vi "GUI Test Chennels.vi"() -> ()   [LabVIEW 2019]
panel:
  out "Vertical Fill Indicator 2":dbl(slide)=5.954198473282443 caption="Температура масла" scale=0.0..10.0
  out "Уровень  масла 2":dbl(slide)=37.72455089820359 caption="Уровень  масла" scale=0.0..100.0
  out "Vertical Fill Indicator":dbl(slide)=5.954198473282443 caption="Температура масла" scale=0.0..10.0
  out "Уровень  масла":dbl(slide)=37.72455089820359 scale=0.0..100.0
  out "DI 17":bool caption="Источник\nпитания 24 В"
  out "DI 9":bool caption="Реле контроля фаз \nКонтактор"
  out "DI 11":bool caption="QF5"
  out "DI 10":bool caption="QF4"
  out "DI 8":bool caption="QF3"
  out "DI 7":bool caption="QF2"
  out "DI 6":bool caption="QF1"
  out "DI 5":bool caption="Автомат"
  out "DI 4":bool caption="Контактор"
  out "DI 3":bool caption="Автомат"
  out "DI 2":bool caption="Контактор"
  out "DI 1":bool caption="Автомат"
  out "DI 0":bool caption="Контактор"
  in  "AO 1":dbl(slide)=1.0 caption="AO 0" scale=0.0..10.0
  in  "AO 0":dbl(slide)=1.0 scale=0.0..10.0
  in  "DO 16":bool caption="KP17"
  in  "DO 15":bool caption="KP16"
  in  "DO 14":bool caption="KP15"
  in  "DO 13":bool caption="KP14"
  in  "DO 12":bool caption="KP13"
  in  "DO 11":bool caption="KP12"
  in  "DO 10":bool caption="KP11"
  in  "DO 9":bool caption="KP10"
  in  "DO 8":bool caption="KP9"
  in  "DO 7":bool caption="KP8"
  in  "DO 6":bool caption="KP7"
  in  "DO 5":bool caption="KP6"
  in  "DO 4":bool caption="KP5"
  in  "DO 3":bool caption="KP4"
  in  "DO 2":bool caption="KP3 [DO 2]"
  in  "DO 1":bool caption="KP2 [DO 1]"
  in  "DO 0":bool caption="KP1 [DO 0]"
  out "DI 16":bool caption="Переключатель ручное/авто SA1"
  out "DI 15":bool caption="Кнопка аварийной остановки SB4"
  out "DI 14":bool caption="Кнопка остановки SB3"
  out "DI 13":bool caption="Кнопка запуска SB2"
  out "DI 12":bool caption="Кнопка сброса ошибки SB1"
  out "Gauge 11":dbl(knob) caption="Датчик давления в линии \nизмерения утечек" scale=0.0..10.0
  out "Gauge 10":dbl(knob) caption="Давление  в  линии подачи \nвоздуха после БПВ" scale=0.0..10.0
  out "Gauge 9":dbl(knob) caption="Давление  в  линии подачи \nвоздуха в БПВ" scale=0.0..10.0
  out "Gauge 8":dbl(knob) caption="Давление в камере" scale=0.0..10.0
  out "Gauge 7":dbl(knob) caption="Давление в образце" scale=0.0..10.0
  out "Gauge 6":dbl(knob) caption="Давление после насоса ВД" scale=0.0..10.0
  # "Проверка каналов"
  # "Панель гидравлическая"
  # "Реле"
  # "Гидростанция очистки и охлаждения"
  # "Насоса перекачки \nв бак подачи"
  # "PUMP1"
  # "PUMP0"
  # "Гидростанция подачи масла"
  # "Кнопки"
  # "Автоматы"
  # "PUMP2"
  # "Управление  подачей давления в насос ВД"
  # "Ethernet Devices"
  # "Регулировка низкого давления в линии подачи масла в насос ВД и напрямую в узел образца"
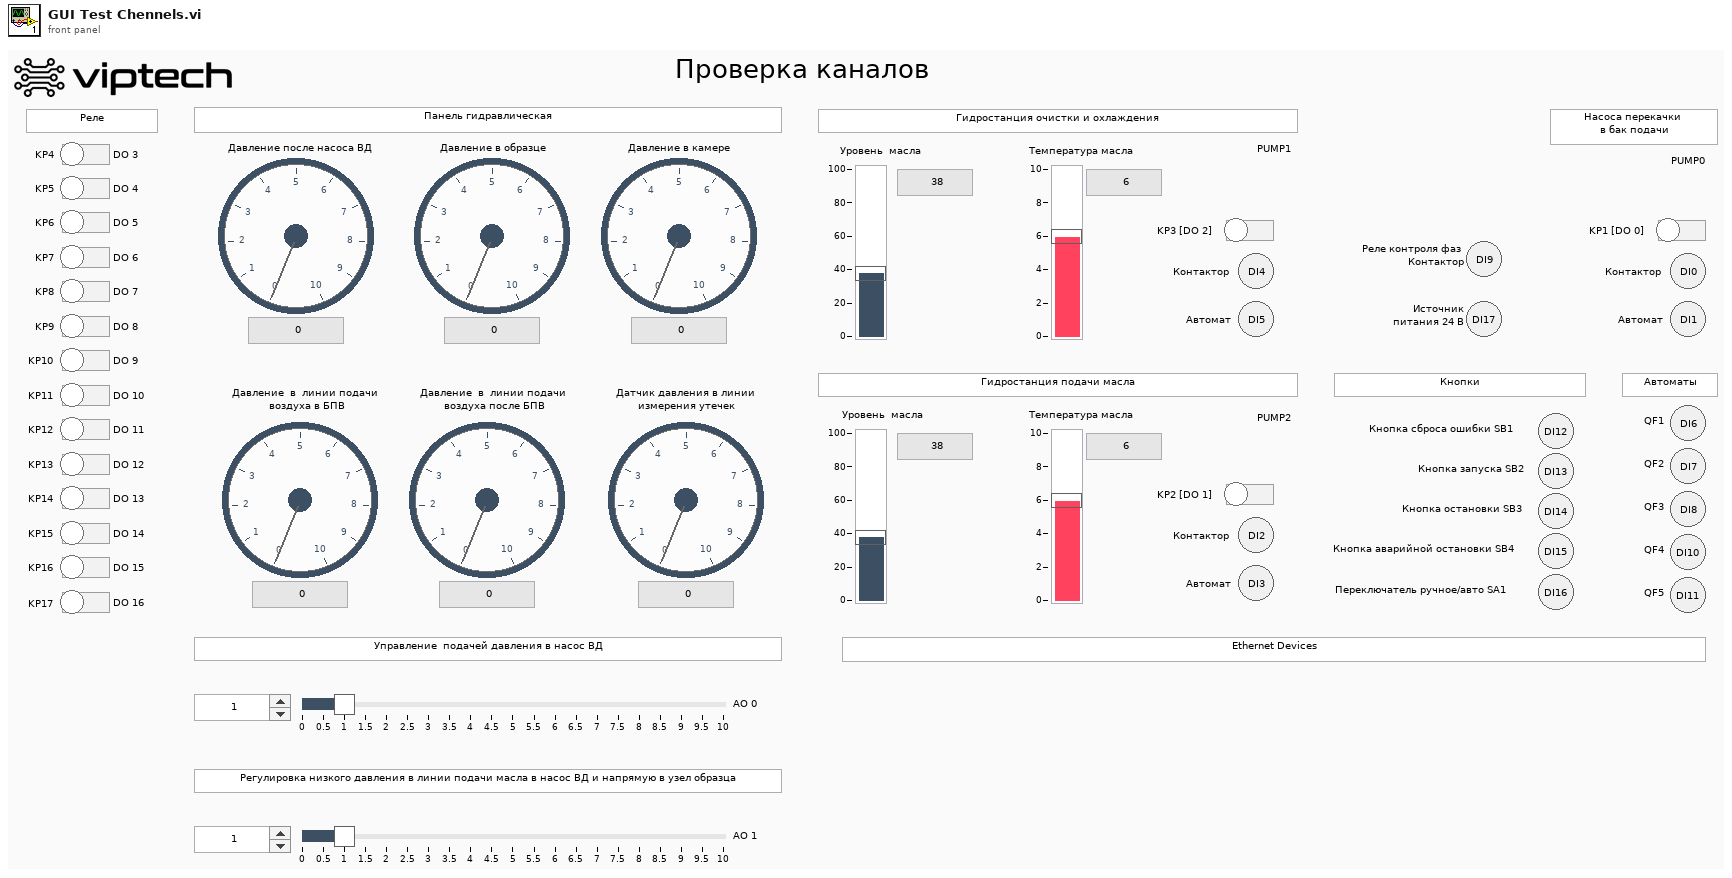
[diagram p1: front panel]
types:
  T1 = enum32{"Invalid", "Standard", "Closed", "Hidden", "Minimized", "Maximized"}
  T2 = enum32{"invalid app kind", "Development System", "Run Time System", "Student Edition", "Embedded LabVIEW", "Evaluation", "Custom"}
  T3 = cluster{"Core":cluster{"Current VI Reference":refnum<vi>, "Close Panel on Exit?":bool}, "Your Boolean data":bool, "Your string data":string}
  T4 = cluster{"Current VI Reference":refnum<vi>, "Close Panel on Exit?":bool}
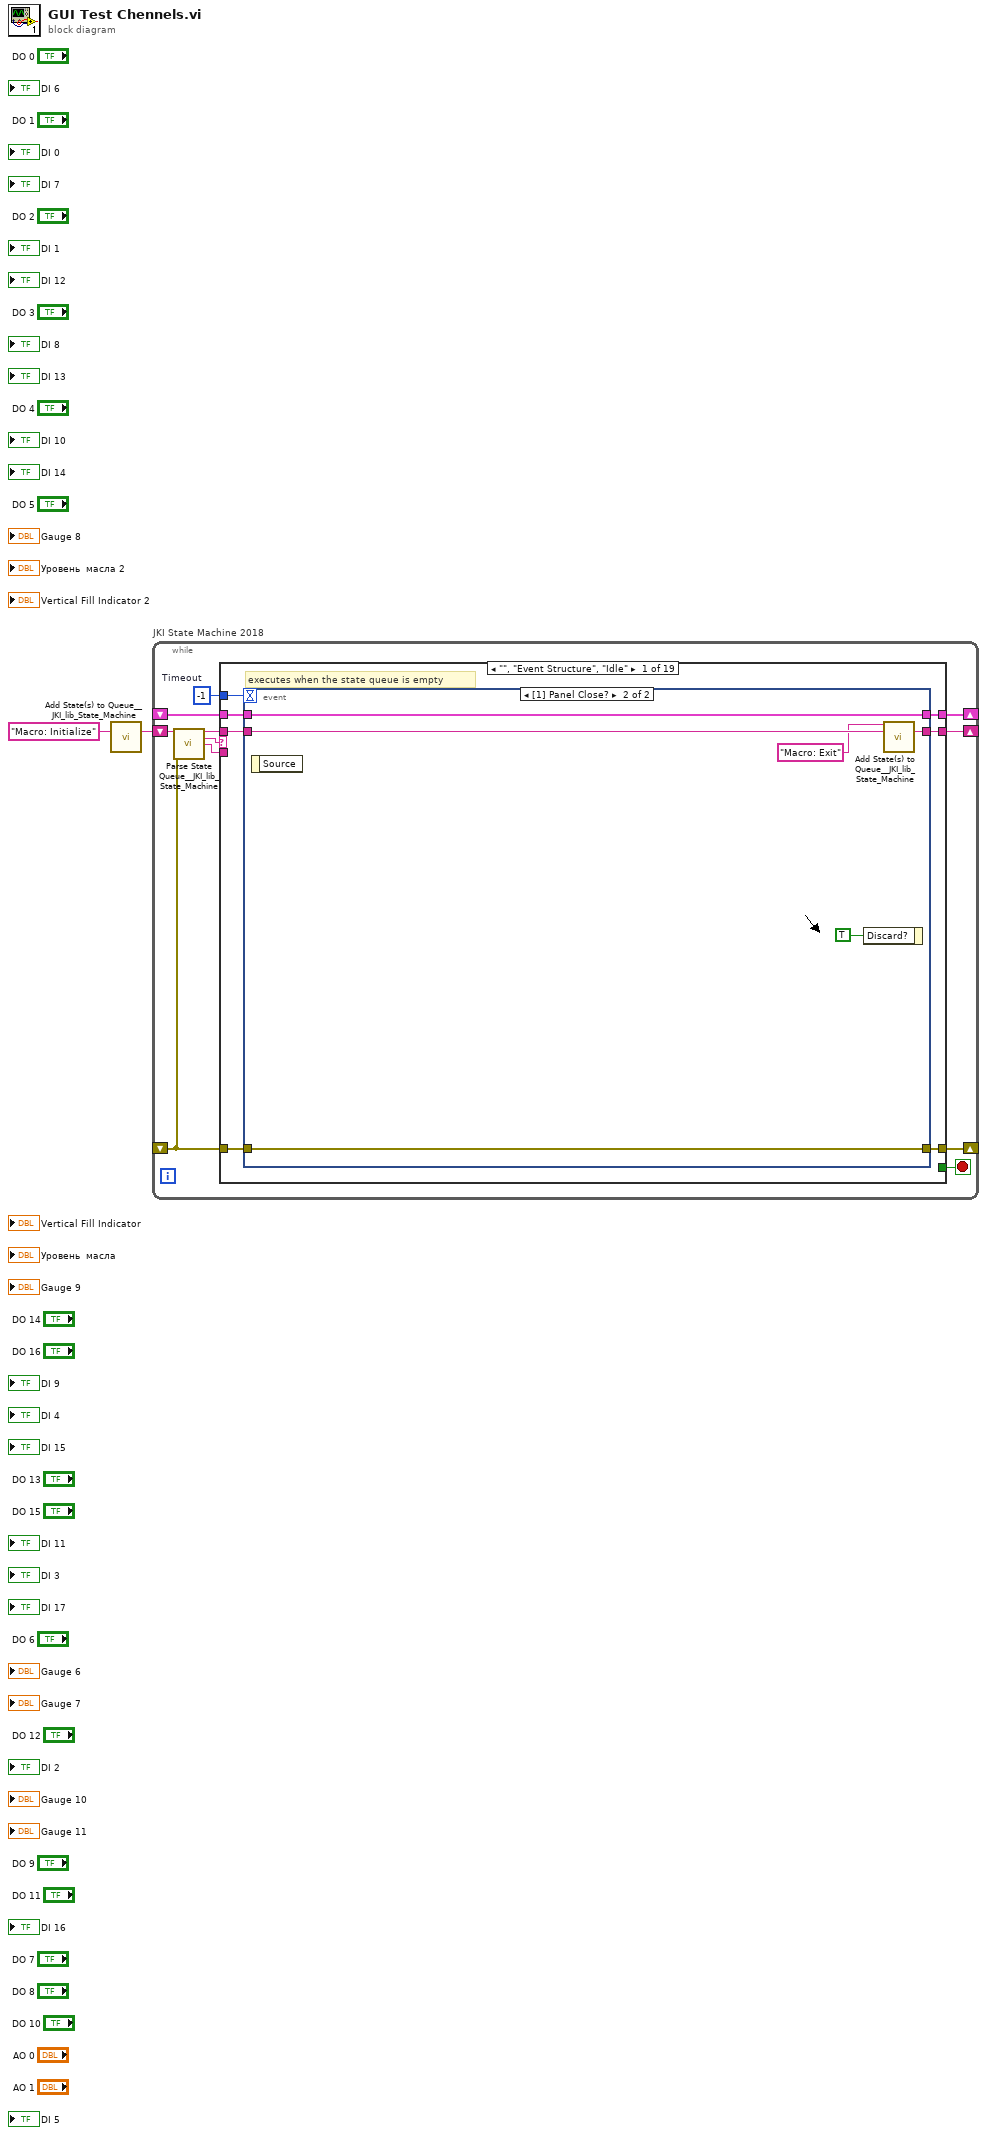
[diagram p0: block diagram]
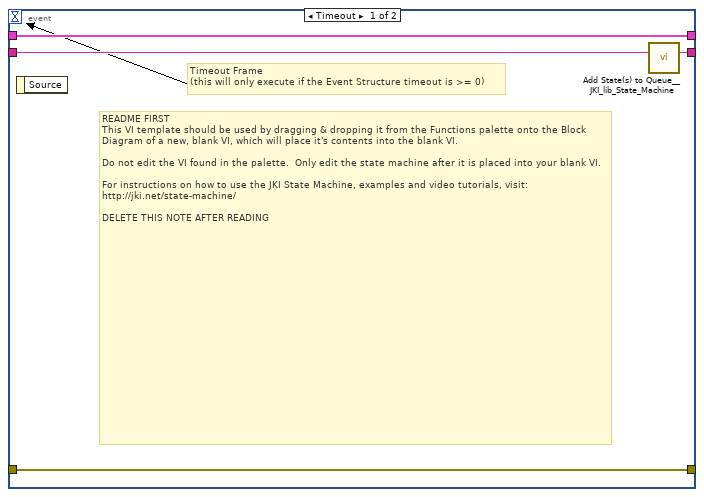
[diagram p2: hidden frame]
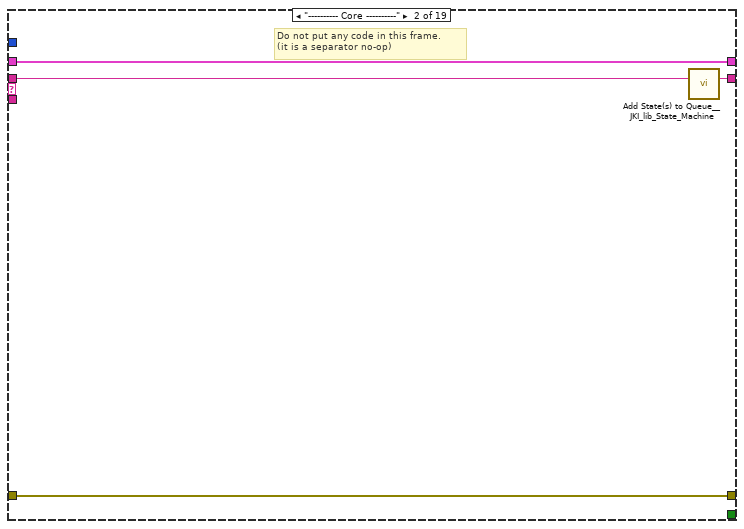
[diagram p3: hidden frame]
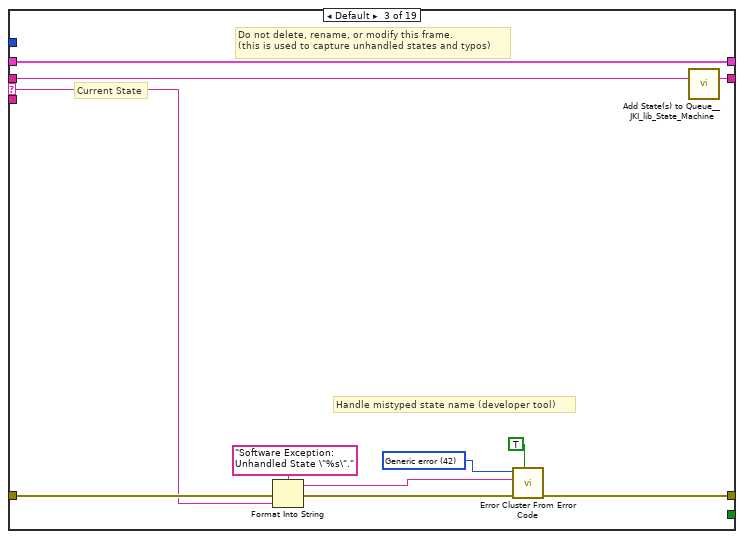
[diagram p4: hidden frame]
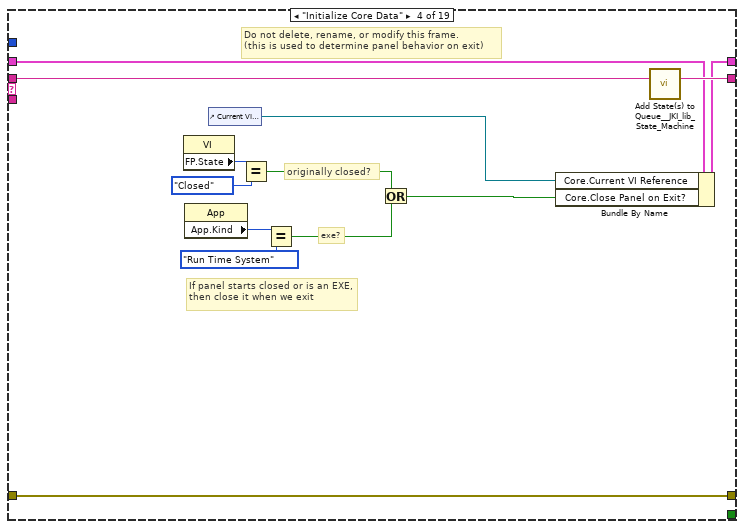
[diagram p5: hidden frame]
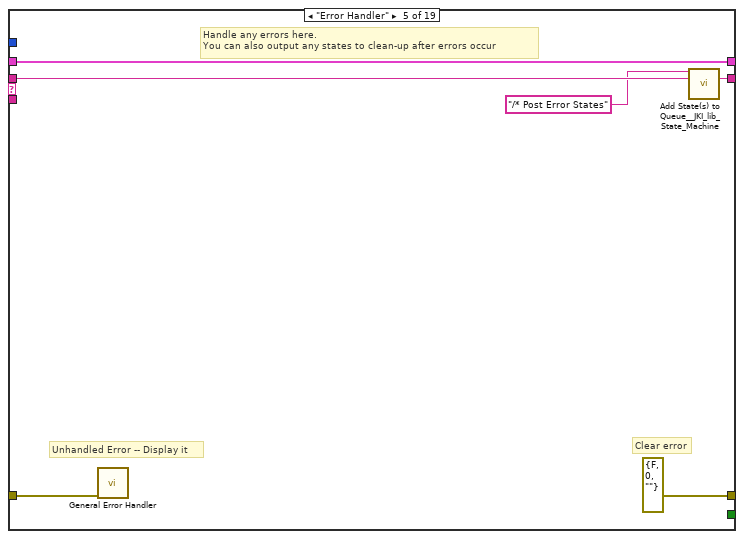
[diagram p6: hidden frame]
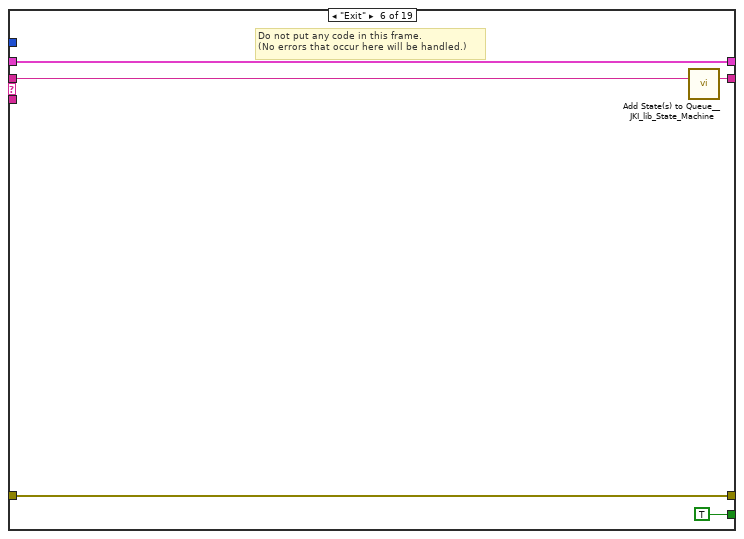
[diagram p7: hidden frame]
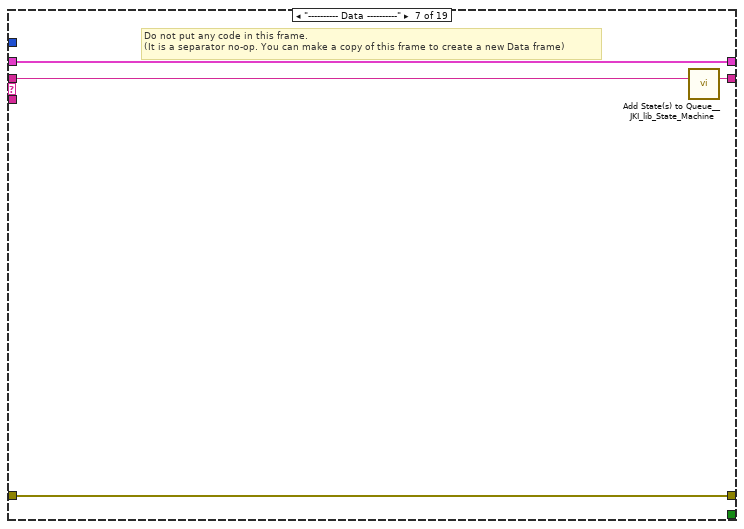
[diagram p8: hidden frame]
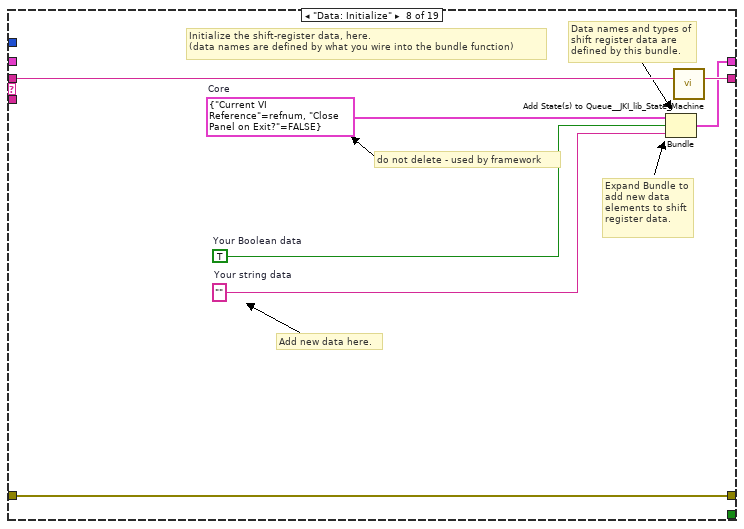
[diagram p9: hidden frame]
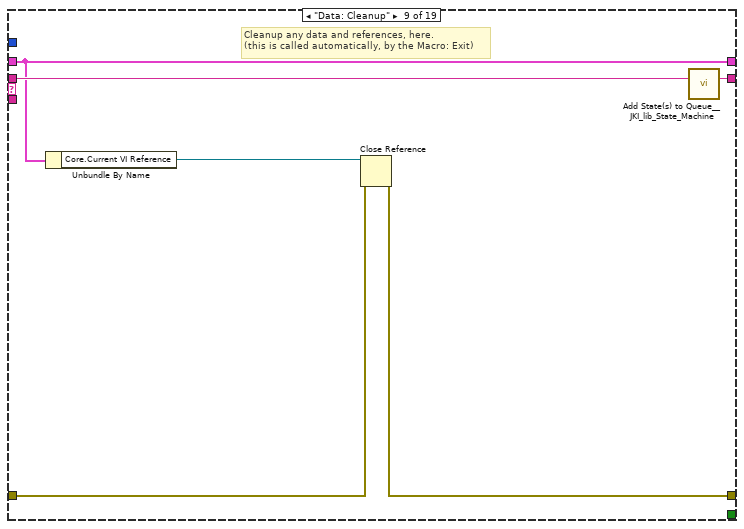
[diagram p10: hidden frame]
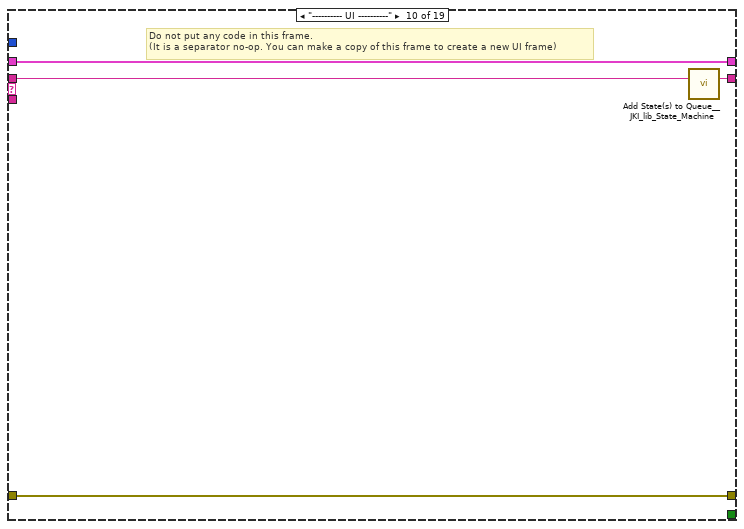
[diagram p11: hidden frame]
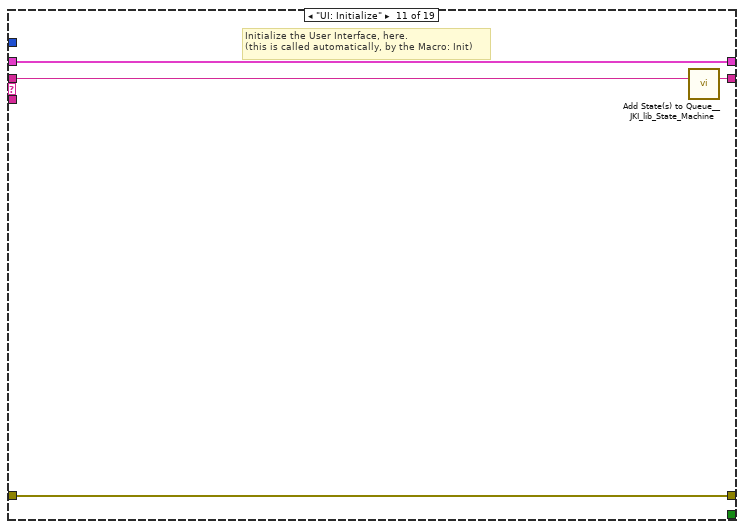
[diagram p12: hidden frame]
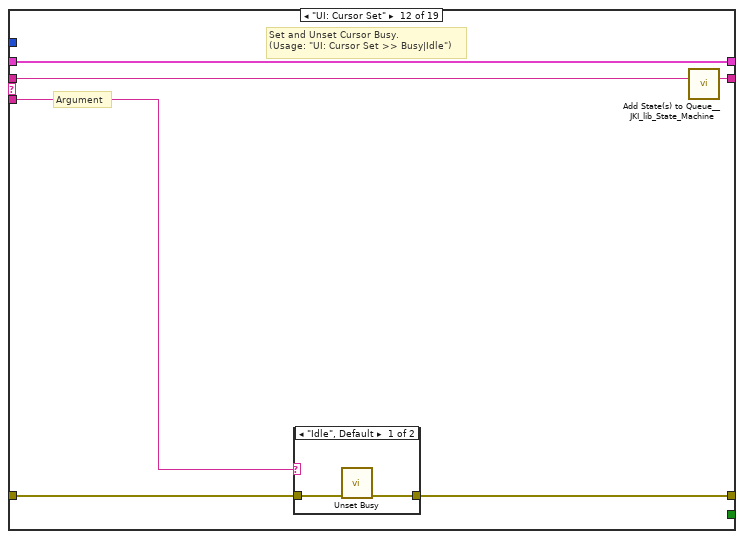
[diagram p13: hidden frame]
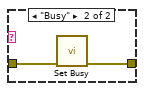
[diagram p14: hidden frame]
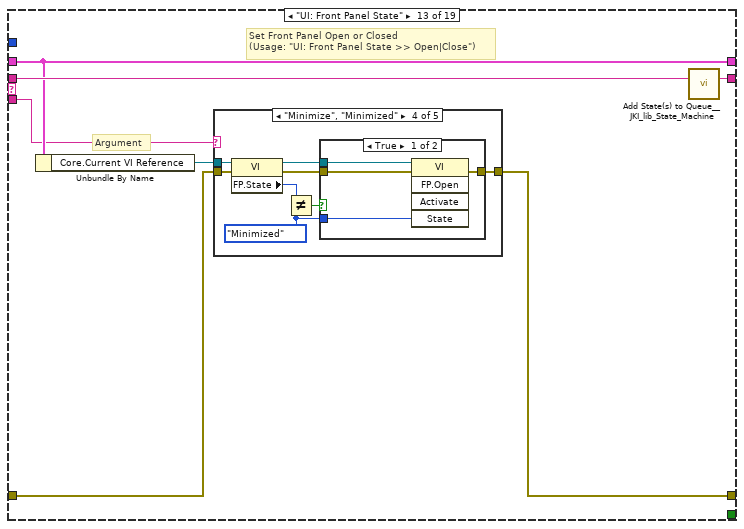
[diagram p15: hidden frame]
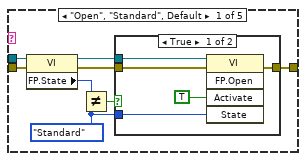
[diagram p16: hidden frame]
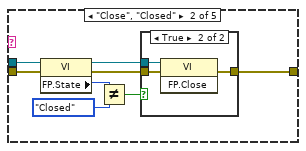
[diagram p18: hidden frame]
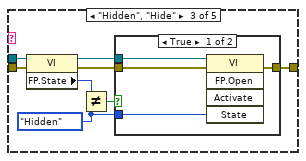
[diagram p20: hidden frame]
diagram:
  n1 = call <vilib>:"Add State(s) to Queue__JKI_lib_State_Machine.vi"("State(s) in (\"\")"="Macro: Initialize") -> ("States Out"=w2:string)  [unwired: 14 in]
  n2 = while "JKI State Machine 2018" {
    shift-right: [w6] -> _
    shift-left: _ -> [w5]
    shift-right: [w9] -> _
    shift-left: _ -> [w3]
    shift-right: [w8] -> _
    shift-left: w2 -> [w10]
    stop <- w7 stop-if-true
    w4 = -1  # Timeout
    n3 = call <vilib>:"Parse State Queue__JKI_lib_State_Machine.vi"("State Queue"=w10, "Error In (no error)"=w3) -> ("Remaining States"=w12:string, "Current State"=w13:string, "Arguments"=w11:string)  [unwired: 11 in]
    n4 = case shown="\"\", \"Event Structure\", \"Idle\"" w13 {
      selector: w13 -> [_ _ w35 _ _ _ _ _ _ _ _ _ _ _ _ _ _ _ _]
      tunnel: w12 -> [w20 w34 w39 w58 w64 w69 w73 w80 w86 w90 w94 w100 w111 w180 w185 w195 w199 w203 w207]
      tunnel: w11 -> [_ _ _ _ _ _ _ _ _ _ _ w95 w105 _ _ _ _ _ _]
      tunnel: w5 -> [w18 w31 w37 w51 w61 w67 w70 _ w81 w87 w92 w98 w107 w177 w182 w192 w196 w200 w204]
      tunnel: [w17 w32 w41 w55 errorcluster {"status"=FALSE, "code"=0, "source"=""} ("error out") w66 w71 w77 w82 w88 w91 w96 w108 w178 w183 w193 w197 w201 w205] -> w9
      tunnel: w3 -> [w16 w32 w40 w55 w60 w66 w71 w77 w83 w88 w91 w97 w109 w178 w183 w193 w197 w201 w205]
      tunnel: [w19 w33 w38 w57 w63 w68 w72 w79 w85 w89 w93 w99 w110 w179 w184 w194 w198 w202 w206] -> w8
      tunnel: [_ _ _ _ _ TRUE _ _ _ _ _ _ _ _ _ _ _ _ _] -> w7
      tunnel: [w15 w31 w37 w56 w61 w67 w70 w78 w81 w87 w92 w98 w107 w177 w182 w192 w196 w200 w204] -> w6
      tunnel: w4 -> [w14 _ _ _ _ _ _ _ _ _ _ _ _ _ _ _ _ _ _]
      frame "", "Event Structure", "Idle" {
        # "executes when the state queue is empty"
        n5 = event shown="[1] Panel Close?" {
          selector: _ -> [_ _]
          dyn-events: _ -> [_ _]
          timeout: w14 -> [_ _]
          tunnel: w20 -> [w24 w30]
          tunnel: [w23 w29] -> w19
          tunnel: w18 -> [w21 w27]
          tunnel: [w22 w28] -> w17
          tunnel: w16 -> [w22 w28]
          tunnel: [w21 w27] -> w15
          event Timeout {
            # "README FIRST\nThis VI template should be used by dragging & dropping it from the Functions palette onto the Block Diagram of a new, blank VI, which will place it's contents into the blank VI.\n\nDo not edit the VI found in the palette.  Only edit the state machine after it is placed into your blank VI.\n\nFor instructions on how to use the JKI State Machine, examples and video tutorials, visit:\nhttp://jki.net/state-machine/\n\nDELETE THIS NOTE AFTER READING"
            # "Timeout Frame\n(this will only execute if the Event Structure timeout is >= 0)"
            n6 = event-data() -> ()  [unwired: 1 in, 1 out]
            n7 = call <vilib>:"Add State(s) to Queue__JKI_lib_State_Machine.vi"("State(s) in (\"\")"=w24) -> ("States Out"=w23:string)  [unwired: 14 in]
          }
          event Panel Close? {
            n8 = event-data() -> ()  [unwired: 1 in, 1 out]
            n9 = event-data("Discard?"=TRUE) -> ()  [unwired: 1 in, 1 out]
            n10 = call <vilib>:"Add State(s) to Queue__JKI_lib_State_Machine.vi"("State(s) in Front (\"\")"="Macro: Exit", "State(s) in (\"\")"=w30) -> ("States Out"=w29:string)  [unwired: 13 in]
          }
        }
      }
      frame "---------- Core ----------" {
        # "Do not put any code in this frame.\n(it is a separator no-op)"
        n11 = call <vilib>:"Add State(s) to Queue__JKI_lib_State_Machine.vi"("State(s) in (\"\")"=w34) -> ("States Out"=w33:string)  [unwired: 14 in]
      }
      frame Default {
        w44 = 42 items=["No error", "Argument error", "Memory is full", "Out of zone", "End of file", "File already open", "Generic file I/O error", "File not found", "File permission error", "Disk is full", "Duplicate path", "Too many files open", "System feature not enabled", "Resource file not found", "Cannot add resource", "Resource not found", "Image not found", "Image memory error", "Pen does not exist", "Config type invalid", "Config token not found", "Config parse error", "Config memory error", "Bad external code format", "Bad external code offset", "External code not present", "Null window", "Destroy window error", "Null menu", "Print aborted", "Bad print record", "Print driver error", "Windows error during printing", "Memory error during printing", "Print dialog error", "Generic print error", "Invalid device refnum", "Device not found", "Device parameter error", "Device unit error", "Cannot open device", "Device call aborted", "Generic error", "Cancelled by user", "Object ID too low", "Object ID too high", "Object not in heap", "Unknown heap", "Unknown object (invalid DefProc)", "Unknown object (DefProc not in table)", "Message out of range", "Invalid (null) method", "Unknown message", "Manager call not supported", "Bad address", "Network operation in progress", "Network operation timed out", "Connection is busy", "Network attribute not supported", "Network error", "Address in use", "System out of memory", "Connection aborted", "Connection refused", "Not connected", "Already connected", "Connection closed", "Initialization error (interapplication manager)", "Bad occurrence", "Wait on unbound occurrence handler", "Occurrence queue overflow", "Datalog type conflict", "Unused", "Unrecognized type (interapplication manager)", "Memory corrupt", "Failed to make temporary DLL", "Old CIN version", "Drag socket not found", "Failed to load drop-object", "Failed to register OLE object", "Failed to release OLE object", "Format specifier type mismatch", "Unknown format specifier", "Too few format specifiers", "Too many format specifiers", "Scan failed", "Newer CIN version", "Error converting to variant", "Runtime menu error", "Password tampered", "Variant attribute not found", "Incompatible variant data type", "Event data is not available", "Event Store is not present", "Occurrence is not found", "Event Queue is not created", "Event info is not available", "Refnum passed is NULL", "Error retrieving Class GUID", "Error retrieving CoClass GUID", "Error retrieving TypeLib GUID.", "Bad built application magic bytes.", "Specific driver is different from the specific driver associated with the Logical Name.", "There is no session opened to the class driver.", "Max Error", "MAX - Error with config objects", "MAX - Error loading configuration", "MAX - Group not supported"]
        # "Current State"
        # "Do not delete, rename, or modify this frame.\n(this is used to capture unhandled states and typos)"
        # "Handle mistyped state name (developer tool)"
        n12 = Format Into String(format string="Software Exception: Unhandled State \"%s\"." ("message"), error in=w40, w35) -> (resulting string=w43:string, error out=w42:errorcluster)  [unwired: 1 in]
        n13 = call <vilib>:"Error Cluster From Error Code.vi"("show call chain? (False)"=TRUE, "error in (no error)"=w42, "error message (\"\")"=w43, "error code (0)"=w44) -> ("error out"=w41:errorcluster)  [unwired: 5 in]
        n14 = call <vilib>:"Add State(s) to Queue__JKI_lib_State_Machine.vi"("State(s) in (\"\")"=w39) -> ("States Out"=w38:string)  [unwired: 14 in]
      }
      frame "Initialize Core Data" {
        # "Do not delete, rename, or modify this frame.\n(this is used to determine panel behavior on exit)"
        # "originally closed?"
        # "exe?"
        # "If panel starts closed or is an EXE, then close it when we exit"
        n15 = property class="VI"() -> ("FP.State"=w48:T1)  [unwired: 2 in, 2 out]
        n16 = property class="App"() -> ("App.Kind"=w54:T2)  [unwired: 2 in, 2 out]
        n17 = control-ref of="Current VI Reference"() -> (w49:refnum<vi>)
        n18 = Equal?(x=w48, y=T1."Closed" ("Front Panel Window:State")) -> (x = y?=w46:bool)
        n19 = Equal?(x=w54, y=T2."Run Time System" ("Application:Kind")) -> (x = y?=w52:bool)
        n20 = Or(x=w46, y=w52) -> (x .or. y?=w50:bool)
        n21 = Bundle By Name(cluster=w51, "Core.Current VI Reference"=w49, "Core.Close Panel on Exit?"=w50) -> (w56:T3)
        n22 = call <vilib>:"Add State(s) to Queue__JKI_lib_State_Machine.vi"("State(s) in (\"\")"=w58) -> ("States Out"=w57:string)  [unwired: 14 in]
      }
      frame "Error Handler" {
        # "Unhandled Error -- Display it"
        # "Handle any errors here.\nYou can also output any states to clean-up after errors occur"
        # "Clear error"
        n23 = call <vilib>:"General Error Handler.vi"("error in (no error)"=w60) -> ()  [unwired: 10 in, 5 out]
        n24 = call <vilib>:"Add State(s) to Queue__JKI_lib_State_Machine.vi"("State(s) in Front (\"\")"="/* Post Error States", "State(s) in (\"\")"=w64) -> ("States Out"=w63:string)  [unwired: 13 in]
      }
      frame "Exit" {
        # "Do not put any code in this frame.\n(No errors that occur here will be handled.)"
        n25 = call <vilib>:"Add State(s) to Queue__JKI_lib_State_Machine.vi"("State(s) in (\"\")"=w69) -> ("States Out"=w68:string)  [unwired: 14 in]
      }
      frame "---------- Data ----------" {
        # "Do not put any code in this frame.\n(It is a separator no-op. You can make a copy of this frame to create a new Data frame)"
        n26 = call <vilib>:"Add State(s) to Queue__JKI_lib_State_Machine.vi"("State(s) in (\"\")"=w73) -> ("States Out"=w72:string)  [unwired: 14 in]
      }
      frame "Data: Initialize" {
        w74 = T4 {"Current VI Reference"=refnum, "Close Panel on Exit?"=FALSE}  # Core
        w76 = TRUE  # Your Boolean data
        w75 = ""  # Your string data
        # "do not delete - used by framework"
        # "Expand Bundle to add new data elements to shift register data."
        # "Add new data here."
        # "Data names and types of shift register data are defined by this bundle."
        # "Initialize the shift-register data, here.\n(data names are defined by what you wire into the bundle function)"
        n27 = Bundle("Core"=w74, "Your Boolean data"=w76, "Your string data"=w75) -> (w78:T3)  [unwired: 1 in]
        n28 = call <vilib>:"Add State(s) to Queue__JKI_lib_State_Machine.vi"("State(s) in (\"\")"=w80) -> ("States Out"=w79:string)  [unwired: 14 in]
      }
      frame "Data: Cleanup" {
        # "Cleanup any data and references, here.\n(this is called automatically, by the Macro: Exit)"
        n29 = Unbundle By Name(w81) -> ("Core.Current VI Reference"=w84:refnum<vi>)
        n30 = Close Reference(reference=w84, error in (no error)=w83) -> (error out=w82:errorcluster)
        n31 = call <vilib>:"Add State(s) to Queue__JKI_lib_State_Machine.vi"("State(s) in (\"\")"=w86) -> ("States Out"=w85:string)  [unwired: 14 in]
      }
      frame "---------- UI ----------" {
        # "Do not put any code in this frame.\n(It is a separator no-op. You can make a copy of this frame to create a new UI frame)"
        n32 = call <vilib>:"Add State(s) to Queue__JKI_lib_State_Machine.vi"("State(s) in (\"\")"=w90) -> ("States Out"=w89:string)  [unwired: 14 in]
      }
      frame "UI: Initialize" {
        # "Initialize the User Interface, here.\n(this is called automatically, by the Macro: Init)"
        n33 = call <vilib>:"Add State(s) to Queue__JKI_lib_State_Machine.vi"("State(s) in (\"\")"=w94) -> ("States Out"=w93:string)  [unwired: 14 in]
      }
      frame "UI: Cursor Set" {
        # "Argument"
        # "Set and Unset Cursor Busy.\n(Usage: \"UI: Cursor Set >> Busy|Idle\")"
        n34 = case shown="\"Idle\", Default" w95 {
          tunnel: w97 -> [w102 w104]
          tunnel: [w101 w103] -> w96
          frame "Idle", Default {
            n35 = call <vilib>:"Unset Busy.vi"("error in (no error)"=w102) -> ("error out"=w101:errorcluster)  [unwired: 10 in]
          }
          frame "Busy" {
            n36 = call <vilib>:"Set Busy.vi"("error in (no error)"=w104) -> ("error out"=w103:errorcluster)  [unwired: 9 in, 1 out]
          }
        }
        n37 = call <vilib>:"Add State(s) to Queue__JKI_lib_State_Machine.vi"("State(s) in (\"\")"=w100) -> ("States Out"=w99:string)  [unwired: 14 in]
      }
      frame "UI: Front Panel State" {
        # "Argument"
        # "Set Front Panel Open or Closed\n(Usage: \"UI: Front Panel State >> Open|Close\")"
        n38 = Unbundle By Name(w107) -> ("Core.Current VI Reference"=w106:refnum<vi>)
        n39 = case shown="\"Minimize\", \"Minimized\"" w105 {
          tunnel: w109 -> [w117 w132 w143 w156 w169]
          tunnel: [w119 w133 w145 w158 w171] -> w108
          tunnel: w106 -> [w118 w130 w144 w157 w170]
          frame "Open", "Standard", Default {
            w112 = T1."Standard" ("State")
            n40 = property class="VI"(reference=w118, error in=w117) -> (reference out=w115:refnum<vi>, error out=w116:errorcluster, "FP.State"=w114:T1)
            n41 = Not Equal?(x=w114, y=w112) -> (x != y?=w113:bool)
            n42 = case shown="True" w113 {
              tunnel: [w123 w125] -> w119
              tunnel: w116 -> [w122 w125]
              tunnel: w115 -> [w121 _]
              tunnel: w112 -> [w120 _]
              frame True {
                n43 = invoke class="VI" method="FP.Open"(reference=w121, error in=w122, "Activate"=TRUE, "State"=w120) -> (error out=w123:errorcluster)  [unwired: 1 in, 4 out]
              }
              frame False {
              }
            }
          }
          frame "Close", "Closed" {
            n44 = property class="VI"(reference=w130, error in=w132) -> (reference out=w129:refnum<vi>, error out=w131:errorcluster, "FP.State"=w127:T1)
            n45 = Not Equal?(x=w127, y=T1."Closed" ("Front Panel Window:State")) -> (x != y?=w126:bool)
            n46 = case shown="True" w126 {
              tunnel: [w134 w137] -> w133
              tunnel: w131 -> [w134 w136]
              tunnel: w129 -> [_ w135]
              frame False {
              }
              frame True {
                n47 = invoke class="VI" method="FP.Close"(reference=w135, error in=w136) -> (error out=w137:errorcluster)  [unwired: 1 in, 2 out]
              }
            }
          }
          frame "Hidden", "Hide" {
            w138 = T1."Hidden" ("State")
            n48 = property class="VI"(reference=w144, error in=w143) -> (reference out=w141:refnum<vi>, error out=w142:errorcluster, "FP.State"=w140:T1)
            n49 = Not Equal?(x=w140, y=w138) -> (x != y?=w139:bool)
            n50 = case shown="True" w139 {
              tunnel: [w149 w150] -> w145
              tunnel: w142 -> [w148 w150]
              tunnel: w141 -> [w147 _]
              tunnel: w138 -> [w146 _]
              frame True {
                n51 = invoke class="VI" method="FP.Open"(reference=w147, error in=w148, "State"=w146) -> (error out=w149:errorcluster)  [unwired: 2 in, 4 out]
              }
              frame False {
              }
            }
          }
          frame "Minimize", "Minimized" {
            w151 = T1."Minimized" ("State")
            n52 = property class="VI"(reference=w157, error in=w156) -> (reference out=w154:refnum<vi>, error out=w155:errorcluster, "FP.State"=w153:T1)
            n53 = Not Equal?(x=w153, y=w151) -> (x != y?=w152:bool)
            n54 = case shown="True" w152 {
              tunnel: [w162 w163] -> w158
              tunnel: w155 -> [w161 w163]
              tunnel: w154 -> [w160 _]
              tunnel: w151 -> [w159 _]
              frame True {
                n55 = invoke class="VI" method="FP.Open"(reference=w160, error in=w161, "State"=w159) -> (error out=w162:errorcluster)  [unwired: 2 in, 4 out]
              }
              frame False {
              }
            }
          }
          frame "Maximize", "Maximized" {
            w164 = T1."Maximized" ("State")
            n56 = property class="VI"(reference=w170, error in=w169) -> (reference out=w167:refnum<vi>, error out=w168:errorcluster, "FP.State"=w166:T1)
            n57 = Not Equal?(x=w166, y=w164) -> (x != y?=w165:bool)
            n58 = case shown="True" w165 {
              tunnel: [w175 w176] -> w171
              tunnel: w168 -> [w174 w176]
              tunnel: w167 -> [w173 _]
              tunnel: w164 -> [w172 _]
              frame True {
                n59 = invoke class="VI" method="FP.Open"(reference=w173, error in=w174, "State"=w172) -> (error out=w175:errorcluster)  [unwired: 2 in, 4 out]
              }
              frame False {
              }
            }
          }
        }
        n60 = call <vilib>:"Add State(s) to Queue__JKI_lib_State_Machine.vi"("State(s) in (\"\")"=w111) -> ("States Out"=w110:string)  [unwired: 14 in]
      }
      frame "---------- Macro ----------" {
        # "Do not put any code in this frame.\n(It is a separator no-op. You can make a copy of this frame to create a new Macro frame)"
        n61 = call <vilib>:"Add State(s) to Queue__JKI_lib_State_Machine.vi"("State(s) in (\"\")"=w180) -> ("States Out"=w179:string)  [unwired: 14 in]
      }
      frame "Macro: Initialize" {
        w181 = "Data: Initialize\nInitialize Core Data\nUI: Initialize\nUI: Front Panel State >> Open"  # Data: Initialize Initialize Core Data UI: Initialize UI: Front Panel State >> Open
        # "Initialization Macro\n(This is called once, when the VI starts)"
        n62 = call <vilib>:"Add State(s) to Queue__JKI_lib_State_Machine.vi"("State(s) in Front (\"\")"=w181, "State(s) in (\"\")"=w185) -> ("States Out"=w184:string)  [unwired: 13 in]
      }
      frame "Macro: Exit" {
        # "Exit Macro\n(This is called once, when the VI exits)"
        n63 = Unbundle By Name(w192) -> ("Core.Close Panel on Exit?"=w191:bool)
        n64 = Select(t="UI: Front Panel State >> Close", s=w191, f="") -> (s? t:f=w188:string)
        n65 = call <vilib>:"Add State(s) to Queue__JKI_lib_State_Machine.vi"("State(s) in (\"\")"=w188, "State(s) at Back (\"\")"="Data: Cleanup\nExit") -> ("States Out"=w186:string)  [unwired: 13 in]
        n66 = call <vilib>:"Add State(s) to Queue__JKI_lib_State_Machine.vi"("State(s) in Front (\"\")"=w186, "State(s) in (\"\")"=w195) -> ("States Out"=w194:string)  [unwired: 13 in]
      }
      frame "---------- New Category ----------" {
        # "Template Separator\n(You can make a copy of, or modify, this frame)"
        n67 = call <vilib>:"Add State(s) to Queue__JKI_lib_State_Machine.vi"("State(s) in (\"\")"=w199) -> ("States Out"=w198:string)  [unwired: 14 in]
      }
      frame "New Category: 1" {
        # "Your code here.\n(You can make a copy of, or modify, this frame)"
        n68 = call <vilib>:"Add State(s) to Queue__JKI_lib_State_Machine.vi"("State(s) in (\"\")"=w203) -> ("States Out"=w202:string)  [unwired: 14 in]
      }
      frame "New Category: 2" {
        # "Your code here.\n(You can make a copy of, or modify, this frame)"
        n69 = call <vilib>:"Add State(s) to Queue__JKI_lib_State_Machine.vi"("State(s) in (\"\")"=w207) -> ("States Out"=w206:string)  [unwired: 14 in]
      }
    }
  }
